vi "Write ToD.vi"(8 "error in (no error)":errorcluster, 10 "ToD":timestamp, 11 "Daily in":refnum<class "Daily.lvclass">) -> (0 "error out":errorcluster, 3 "Daily out":refnum<class "Daily.lvclass">)   [LabVIEW 2020, in "Daily.lvclass"]
uses:
  Daily.lvclass
  Daily.lvclass/Daily.ctl
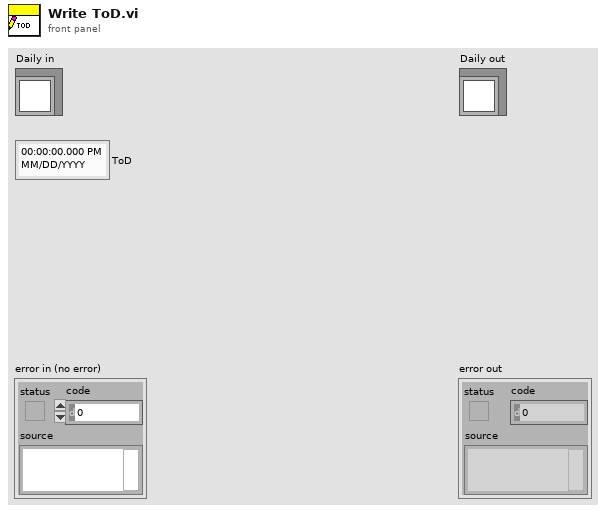
[diagram p1: front panel]
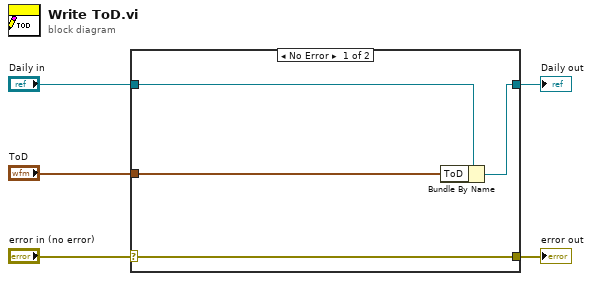
[diagram p0: block diagram]
diagram:
  n1 = case shown="No Error" "error in (no error)" {
    selector: "error in (no error)" -> [w9 w10]
    tunnel: [w9 w10] -> w4
    tunnel: [w7 w11] -> w2
    tunnel: "Daily in" -> [w8 w11]
    tunnel: "ToD" -> [w6 _]
    frame No Error {
      n2 = Bundle By Name(cluster=w8, "ToD"=w6) -> (w7:refnum<class "Daily.lvclass">)
    }
    frame Error {
    }
  }
  "error out" <- w4
  "Daily out" <- w2
